vi "robot control from internet.vi"() -> ()   [LabVIEW 2012, in "Tank Robot.lvrbt"]
uses:
  Tank Robot.lvrbt
  <vilib>/NXT/Subs/MotorXNode.1Servo.ctl
  <vilib>/NXT/Subs/MotorXNode.Servo Type.ctl
  <vilib>/NXT/Subs/MotorXNode.2DCMotor.ctl
  <vilib>/NXT/Subs/MotorXNode.DC Motor Type.ctl
  <vilib>/NXT/NXTIO Xnodes/NXTIONodeSubVIs/TETRIX IO Move Servos.vi
  <vilib>/NXT/Dual Mode Library/Display/drawNumber_float.vi
  <vilib>/NXT/NXTIO Xnodes/NXTIONodeSubVIs/TETRIX IO Move DC Motors.vi
  <vilib>/NXT/Subs/LVHSConnector.ctl
  <vilib>/NXT/NXTIO Xnodes/AddressXNode/NXTIOAddress.xnode
  <vilib>/NXT/NXTIO Xnodes/NXTIOXNode/NXTIO.xnode
panel:
  out "Servo State":dbl
  out "Right":bool
  out "Left":bool
  out "Bottom":bool
  out "Top":bool
  out "Drive State":dbl
  in  "Speed":dbl(slide) scale=0.0..100.0
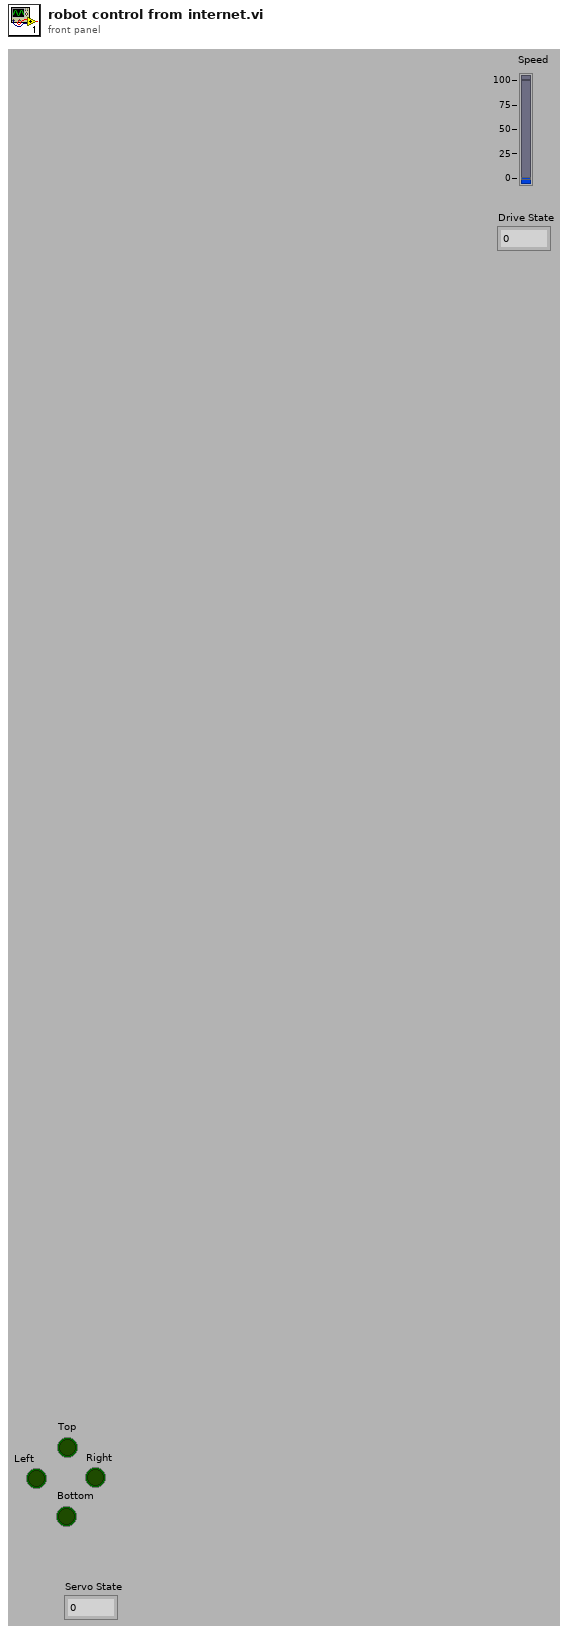
[diagram p1: front panel]
types:
  T1 = typedef "MotorXNode.DC Motor Type.ctl" = enum16{"DC Motor"}
  T2 = cluster{"DC Motor":T1, "Address":i16, "Address":i16}
  T3 = typedef "MotorXNode.Servo Type.ctl" = enum16{"Servo"}
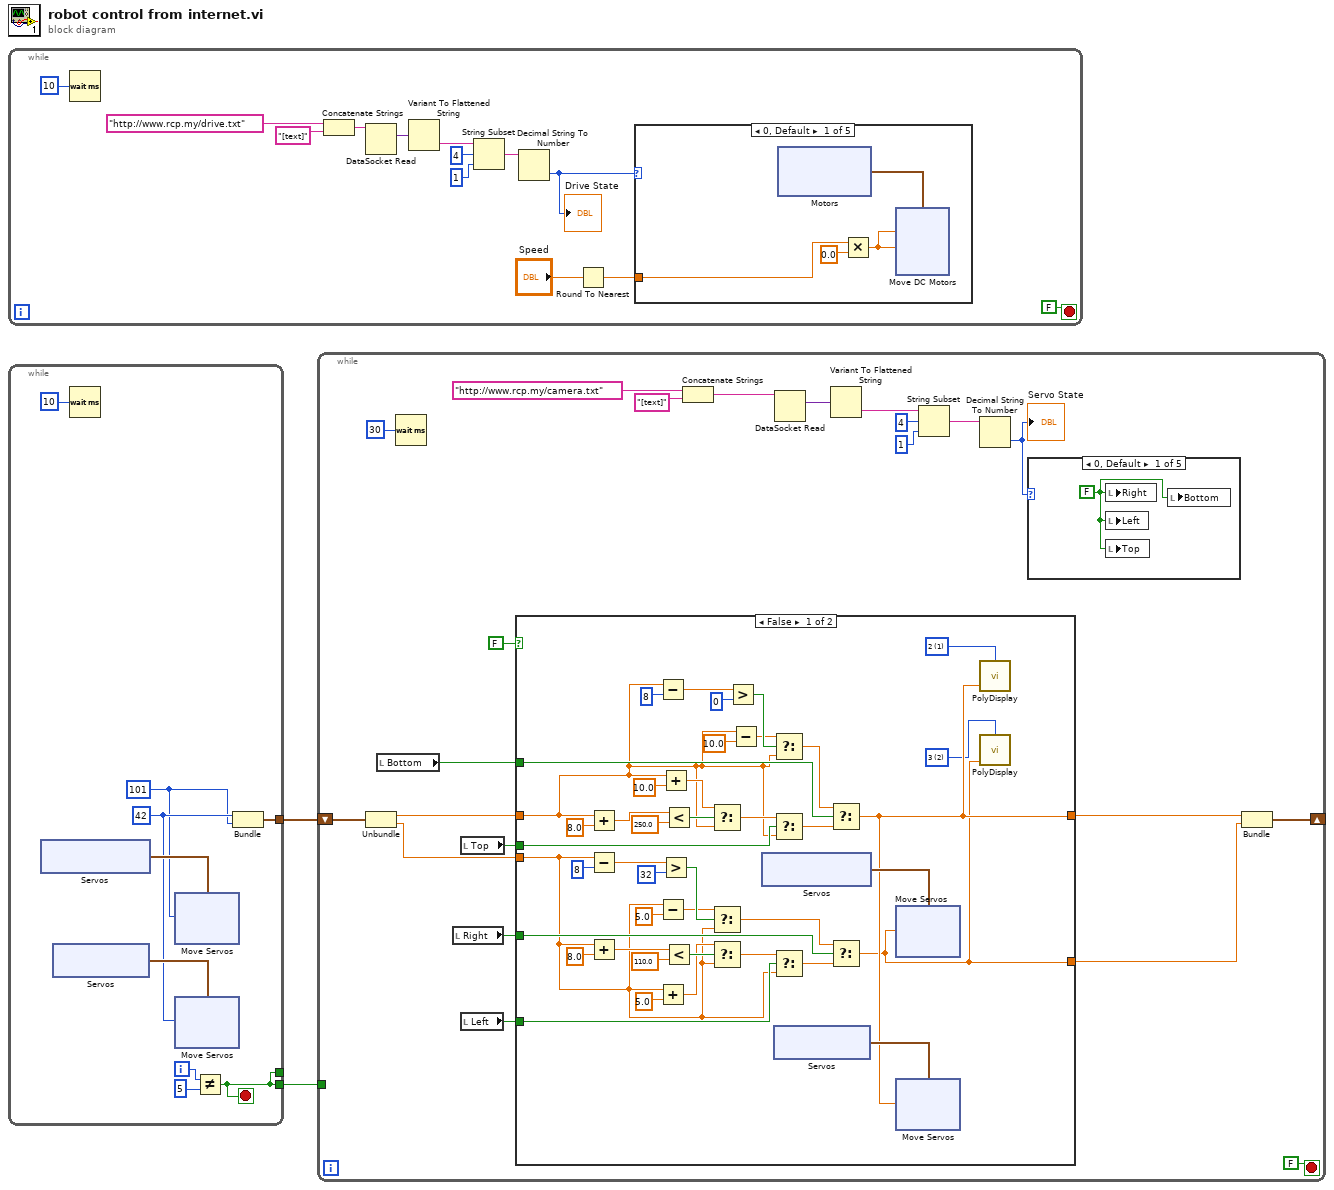
[diagram p0: block diagram]
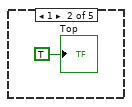
[diagram p2: hidden frame]
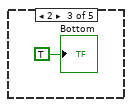
[diagram p3: hidden frame]
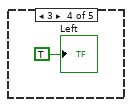
[diagram p4: hidden frame]
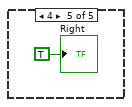
[diagram p5: hidden frame]
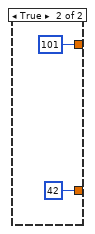
[diagram p6: hidden frame]
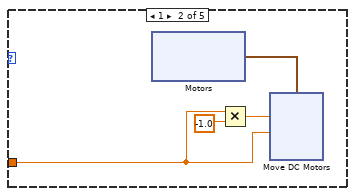
[diagram p7: hidden frame]
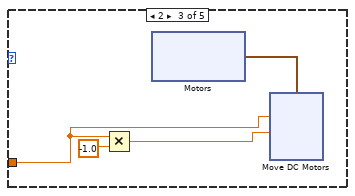
[diagram p8: hidden frame]
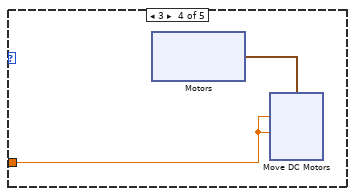
[diagram p9: hidden frame]
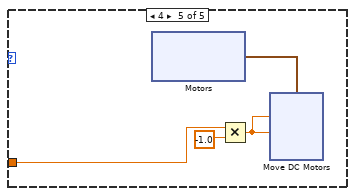
[diagram p10: hidden frame]
diagram:
  n1 = while {
    stop <- FALSE stop-if-true
    n2 = Wait (ms)(milliseconds to wait=u32 10) -> ()  [unwired: 1 out]
    n3 = Concatenate Strings("http://www.rcp.my/drive.txt" ("connection in"), "[text]" ("string")) -> (w13:string)
    n4 = DataSocket Read(11:w13) -> (2:w11:variant)  [unwired: 4 in, 6 out]
    n5 = Variant To Flattened String(Variant=w11) -> (data string=w7:string)  [unwired: 1 out]
    n6 = String Subset(string=w7, offset (0)=4, length (rest)=1 ("length (rest)")) -> (substring=w8:string)
    n7 = Decimal String To Number(string=w8) -> (number=w4:i32)  [unwired: 2 in, 1 out]
    "Drive State" <- w4
    n8 = Round To Nearest(number="Speed") -> (nearest integer value=w6:dbl)
    n9 = case shown="0, Default" w4 {
      tunnel: w6 -> [w18 w31 w46 w61 w76]
      frame 0, Default {
        n10 = xnode "Motors"() -> ("DC Motor"=w19:T2)
        n11 = Multiply(x=w18, y=0.0) -> (x*y=w16:dbl)
        n12 = xnode "Move DC Motors"("Power/Speed 2"=w16, "Power/Speed 1"=w16, "Motors"=w19) -> ()  [unwired: 1 in, 1 out]
      }
      frame 1 {
        n13 = xnode "Motors"() -> ("DC Motor"=w34:T2)
        n14 = Multiply(x=w31, y=-1.0) -> (x*y=w32:dbl)
        n15 = xnode "Move DC Motors"("Power/Speed 2"=w31, "Power/Speed 1"=w32, "Motors"=w34) -> ()  [unwired: 1 in, 1 out]
      }
      frame 2 {
        n16 = Multiply(x=w46, y=-1.0) -> (x*y=w47:dbl)
        n17 = xnode "Motors"() -> ("DC Motor"=w49:T2)
        n18 = xnode "Move DC Motors"("Power/Speed 2"=w47, "Power/Speed 1"=w46, "Motors"=w49) -> ()  [unwired: 1 in, 1 out]
      }
      frame 3 {
        n19 = xnode "Motors"() -> ("DC Motor"=w62:T2)
        n20 = xnode "Move DC Motors"("Power/Speed 2"=w61, "Power/Speed 1"=w61, "Motors"=w62) -> ()  [unwired: 1 in, 1 out]
      }
      frame 4 {
        n21 = xnode "Motors"() -> ("DC Motor"=w77:T2)
        n22 = Multiply(x=w76, y=-1.0) -> (x*y=w74:dbl)
        n23 = xnode "Move DC Motors"("Power/Speed 2"=w74, "Power/Speed 1"=w74, "Motors"=w77) -> ()  [unwired: 1 in, 1 out]
      }
    }
  }
  n24 = while {
    tunnel: [w89] -> _
    tunnel: [w90] -> w1
    tunnel: [w89] -> w2
    i -> [w97]
    stop <- w89 stop-if-true
    w91 = u8 101 ("Position 1")
    w92 = u8 42 ("Position 1")
    n25 = xnode "Servos"() -> ("Servo"=w93:cluster{"Servo":T3, "Address":i16})
    n26 = xnode "Servos"() -> ("Servo"=w94:cluster{"Servo":T3, "Address":i16})
    n27 = Wait (ms)(milliseconds to wait=u32 10) -> ()  [unwired: 1 out]
    n28 = xnode "Move Servos"("Position 1"=w91, "Servos"=w93) -> ()  [unwired: 1 in, 1 out]
    n29 = xnode "Move Servos"("Position 1"=w92, "Servos"=w94) -> ()  [unwired: 1 in, 1 out]
    n30 = Not Equal?(x=w97, y=5) -> (x != y?=w89:bool)
    n31 = Bundle("Position 1"=w92, "Position 1"=w91) -> (w90:cluster{"Position 1":u8, "Position 1":u8})  [unwired: 1 in]
  }
  n32 = while {
    shift-right: [w131] -> _
    shift-left: w1 -> [w130]
    tunnel: w2 -> [_]
    stop <- FALSE stop-if-true
    n33 = Unbundle(w130) -> ("Position 1"=w134:dbl, "Position 1"=w133:dbl)
    n34 = local read "Bottom"() -> (w117:bool)
    n35 = Wait (ms)(milliseconds to wait=u32 30) -> ()  [unwired: 1 out]
    n36 = local read "Right"() -> (w118:bool)
    n37 = local read "Top"() -> (w116:bool)
    n38 = local read "Left"() -> (w132:bool)
    n39 = case shown="False" FALSE {
      tunnel: w117 -> [w176 _]
      tunnel: w116 -> [w175 _]
      tunnel: w134 -> [w167 _]
      tunnel: [w146 101] -> w136
      tunnel: w118 -> [w149 _]
      tunnel: w132 -> [w148 _]
      tunnel: w133 -> [w147 _]
      tunnel: [w144 42] -> w135
      frame False {
        w143 = i16 2 items=["1", "2", "3", "4", "5", "6", "7", "8"] ("Line")
        w145 = i16 1 items=["1", "2", "3", "4", "5", "6", "7", "8"] ("Line")
        n40 = Add(x=w167, y=8.0) -> (x+y=w173:dbl)
        n41 = Subtract(x=w147, y=u8 8) -> (x-y=w163:dbl)
        n42 = Add(x=w147, y=8.0) -> (x+y=w156:dbl)
        n43 = Subtract(x=w167, y=u8 8) -> (x-y=w182:dbl)
        n44 = Subtract(x=w147, y=5.0) -> (x-y=w160:dbl)
        n45 = Add(x=w147, y=5.0) -> (x+y=w153:dbl)
        n46 = Add(x=w167, y=10.0) -> (x+y=w170:dbl)
        n47 = Greater?(x=w163, y=u8 32) -> (0:w161:bool)
        n48 = Less?(x=w173, y=250.0) -> (x < y?=w171:bool)
        n49 = Less?(x=w156, y=110.0) -> (x < y?=w154:bool)
        n50 = Select(t=w170, s=w171, f=w167) -> (s? t:f=w168:dbl)
        n51 = Select(t=w160, s=w161, f=w147) -> (s? t:f=w158:dbl)
        n52 = Select(t=w153, s=w154, f=w147) -> (s? t:f=w151:dbl)
        n53 = Greater?(x=w182, y=u8 0) -> (0:w180:bool)
        n54 = Subtract(x=w167, y=10.0) -> (x-y=w179:dbl)
        n55 = xnode "Servos"() -> ("Servo"=w165:cluster{"Servo":T3, "Address":i16})
        n56 = Select(t=w179, s=w180, f=w167) -> (s? t:f=w177:dbl)
        n57 = Select(t=w168, s=w175, f=w167) -> (s? t:f=w166:dbl)
        n58 = Select(t=w151, s=w148, f=w147) -> (s? t:f=w150:dbl)
        n59 = xnode "Servos"() -> ("Servo"=w184:cluster{"Servo":T3, "Address":i16})
        n60 = Select(t=w177, s=w176, f=w166) -> (s? t:f=w146:dbl)
        n61 = Select(t=w158, s=w149, f=w150) -> (s? t:f=w144:dbl)
        n62 = xnode "Move Servos"("Position 1"=w144, "Servos"=w165) -> ()  [unwired: 1 in, 1 out]
        n63 = xnode "Move Servos"("Position 1"=w146, "Servos"=w184) -> ()  [unwired: 1 in, 1 out]
        n64 = call-poly <vilib>:"PolyDisplay.vi"("number"=w146, "Line"=w145) -> ()  [unwired: 2 in, 1 out]
        n65 = call-poly <vilib>:"PolyDisplay.vi"("number"=w144, "Line"=w143) -> ()  [unwired: 2 in, 1 out]
      }
      frame True {
      }
    }
    n66 = Concatenate Strings("http://www.rcp.my/camera.txt" ("connection in"), "[text]" ("string")) -> (w126:string)
    n67 = DataSocket Read(11:w126) -> (2:w125:variant)  [unwired: 4 in, 6 out]
    n68 = Variant To Flattened String(Variant=w125) -> (data string=w121:string)  [unwired: 1 out]
    n69 = String Subset(string=w121, offset (0)=4, length (rest)=1 ("length (rest)")) -> (substring=w122:string)
    n70 = Decimal String To Number(string=w122) -> (number=w120:i32)  [unwired: 2 in, 1 out]
    "Servo State" <- w120
    n71 = case shown="0, Default" w120 {
      frame 0, Default {
        w138 = FALSE ("Right")
        n72 = local write "Right"(w138) -> ()
        n73 = local write "Left"(w138) -> ()
        n74 = local write "Top"(w138) -> ()
        n75 = local write "Bottom"(w138) -> ()
      }
      frame 1 {
        "Top" <- TRUE ("Top")
      }
      frame 2 {
        "Bottom" <- TRUE ("Bottom")
      }
      frame 3 {
        "Left" <- TRUE ("Left")
      }
      frame 4 {
        "Right" <- TRUE ("Right")
      }
    }
    n76 = Bundle("Position 1"=w136, "Position 1"=w135) -> (w131:cluster{"Position 1":dbl, "Position 1":dbl})  [unwired: 1 in]
  }
